vi "Command Engine.vi"(8 "error in (no error)":errorcluster, 10 "Parameters":T1 {"Compiled"."External Channels"."Channels" format="%.0x"; "Compiled"."External Channels"."Triggers" format="%.0x"}, 11 "Global Variables":T12) -> (0 "error out":errorcluster)   [LabVIEW 2015, in "Instrument Addon Engine.lvlib"]
uses:
  Instrument Addon Engine.lvlib
  Types/Engine State Variables.ctl
  <vilib>/NI/NIVS Inline Async API/_VS Inline Async API/Process/Process.lvclass
  <vilib>/NI/NIVS Addon Network Comm/Engine/VeriStand Comm.lvclass
  <vilib>/NI/NIVS Inline Async API/_Data Access Engine/Data Access Engine/Types/Write.DVR.ctl
  <vilib>/NI/NIVS Inline Async API/_Data Access Engine/Access Type Classes/Write/Write.lvclass
  <vilib>/NI/NIVS Inline Async API/_Data Access Engine/Data Access Engine/Types/Read.DVR.ctl
  <vilib>/NI/NIVS Inline Async API/_Data Access Engine/Access Type Classes/Read/Read.lvclass
  <vilib>/NI/NIVS Inline Async API/_Data Access Engine/Data Access Engine/Types/ReadWrite.DVR.ctl
  <vilib>/NI/NIVS Inline Async API/_Data Access Engine/Access Type Classes/ReadWrite/ReadWrite.lvclass
  Types/Commands RT Configuration Cluster.ctl
  Protocols.lvlibp/Protocol Parent/Protocol Parent.lvclass
  Shared/Types/Compiled Settings.ctl
  Shared/Types/Command Parameters.ctl
  Shared/Types/Linked Channel Cluster.ctl
  Shared/Types/Response RT Configuration Cluster.ctl
  Shared/Types/Response Parameters.ctl
  Shared/Types/Response Wait Type.ctl
  Shared/Types/Message Parameters.ctl
  Shared/Types/Message Generation Type.ctl
  Shared/Types/External Trigger Refs.ctl
  <vilib>/NI Veristand/Custom Device API/Data Reference.ctl
  Protections.lvlibp/Parent Protection/Protection.lvclass
  <vilib>/NI/NIVS Inline Async API/_Data Access Engine/Access Type Classes/ReadWrite/ReadWrite.lvclass/ReadWrite.ctl
  <vilib>/NI/NIVS Inline Async API/_Data Access Engine/Access Type Classes/Read/Read.lvclass/Read.ctl
  <vilib>/NI/NIVS Inline Async API/_Data Access Engine/Access Type Classes/Write/Write.lvclass/Write.ctl
  <vilib>/NI/NIVS Inline Async API/_VS Inline Async API/Process/Process.lvclass/Process.ctl
  Determine Trigger.vi
  <vilib>/NI/NIVS Inline Async API/_Data Access Engine/Data Access Engine/Methods/Data.Processes.Execute.vi
  <vilib>/NI/NIVS Inline Async API/_Data Access Engine/Data Access Engine/Methods/ReadWrite.Data.Read.vi
  <vilib>/NI/NIVS Inline Async API/_Data Access Engine/Data Access Engine/Methods/Read.Data.vi
  Format Instrument String Command.vi
  <vilib>/NI/NIVS Inline Async API/_Data Access Engine/Data Access Engine/Methods/Write.Data.vi
  <vilib>/NI/NIVS Inline Async API/_Data Access Engine/Data Access Engine/Methods/ReadWrite.Data.Reset.vi
  <vilib>/NI/NIVS Inline Async API/_VS Inline Async API/Error Handling Process/SubVIs/Error.ConvertArray.vi
  <vilib>/NI/NIVS Inline Async API/_Data Access Engine/Access Type Classes/ReadWrite/ReadWrite.ProcessData.Read.vi
  <vilib>/NI/NIVS Inline Async API/_Data Access Engine/Access Type Classes/Read/Read.ProcessData.vi
  Format Numeric to String.vi
  <vilib>/NI/NIVS Inline Async API/_Data Access Engine/Access Type Classes/Write/Write.ProcessData.vi
  <vilib>/NI/NIVS Inline Async API/_Data Access Engine/Access Type Classes/ReadWrite/ReadWrite.ProcessData.Reset.vi
  Get Wait Value from Channel.vi
  Send Instrument String Command.vi
  Wait on Instrument String Response.vi
  Format Instrument String Response.vi
  <vilib>/NI/AMC/AMC.lvlib
  Shared/Instrument Addon Shared.lvlib
  <vilib>/NI VeriStand/Custom Device API/Custom Device API.lvlib
  <vilib>/NI/NIVS Inline Async API/_Data Access Engine/Data Access Engine/Data Access Engine.lvclass
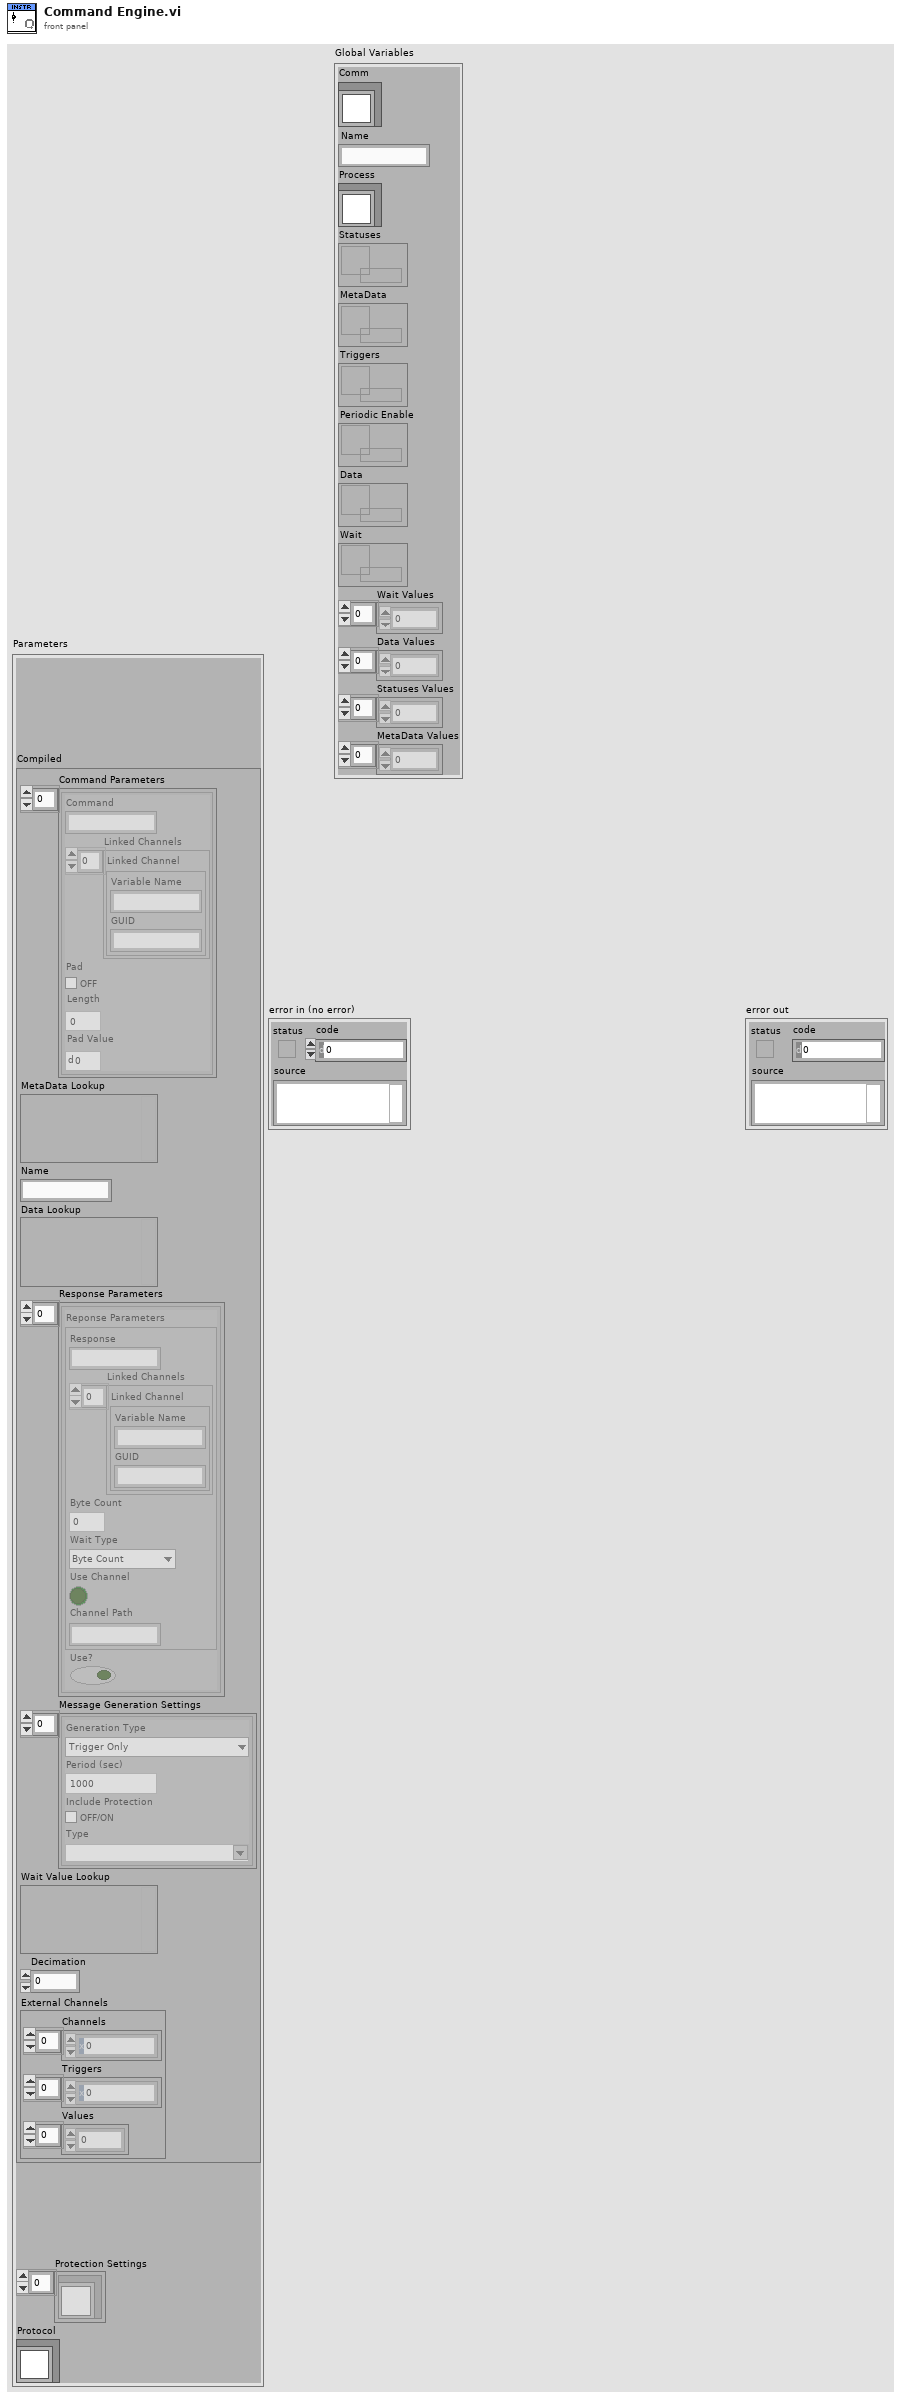
[diagram p1: front panel]
types:
  T1 = typedef "Instrument Addon Engine.lvlib/Commands RT Configuration Cluster.ctl" = cluster{"Compiled":T2, "Protection Settings":refnum<class "Protection.lvclass">[], "Protocol":refnum<class "Protocol Parent.lvclass">}
  T2 = typedef "Instrument Addon Shared.lvlib/Compiled Settings.ctl" = cluster{"Command Parameters":T3[], "MetaData Lookup":variant, "Name":string, "Data Lookup":variant, "Response Parameters":T5[], "Message Generation Settings":T8[], "Wait Value Lookup":variant, "Decimation":u32, "External Channels":T10}
  T3 = typedef "Instrument Addon Shared.lvlib/Command Parameters.ctl" = cluster{"Command":string, "Linked Channels":T4[], "Pad":bool, "Length":u32, "Pad Value":u8}
  T4 = typedef "Instrument Addon Shared.lvlib/Linked Channel Cluster.ctl" = cluster{"Variable Name":string, "GUID":string}
  T5 = typedef "Instrument Addon Shared.lvlib/Response RT Configuration Cluster.ctl" = cluster{"Reponse Parameters":T6, "Use?":bool}
  T6 = typedef "Instrument Addon Shared.lvlib/Response Parameters.ctl" = cluster{"Response":string, "Linked Channels":T4[], "Type Value":dbl, "Wait Type":T7, "Use Channel":bool, "Channel Path":string}
  T7 = typedef "Instrument Addon Shared.lvlib/Response Wait Type.ctl" = enum16{"Byte Count", "Wait sec"}
  T8 = typedef "Instrument Addon Shared.lvlib/Message Parameters.ctl" = cluster{"Generation Type":T9, "Period":dbl, "Include Protection":bool, "Type":string}
  T9 = typedef "Instrument Addon Shared.lvlib/Message Generation Type.ctl" = enum16{"Trigger Only", "Periodic & Trigger"}
  T10 = typedef "Instrument Addon Shared.lvlib/External Trigger Refs.ctl" = cluster{"Channels":T11[], "Triggers":T11[], "Values":dbl[]}
  T11 = typedef "Custom Device API.lvlib/Data Reference.ctl" = i32
  T12 = typedef "Instrument Addon Engine.lvlib/Engine State Variables.ctl" = cluster{"Comm":refnum<class "VeriStand Comm.lvclass">, "Name":string, "Process":refnum<class "Process.lvclass">, "Statuses":T13, "MetaData":T14, "Triggers":T15, "Periodic Enable":T14, "Data":T13, "Wait":T14, "Wait Values":dbl[], "Data Values":dbl[], "Statuses Values":dbl[], "MetaData Values":dbl[]}
  T13 = typedef "Data Access Engine.lvlib/Data Access Engine.lvclass/Write.DVR.ctl" = refnum<data-value>
  T14 = typedef "Data Access Engine.lvlib/Data Access Engine.lvclass/Read.DVR.ctl" = refnum<data-value>
  T15 = typedef "Data Access Engine.lvlib/Data Access Engine.lvclass/ReadWrite.DVR.ctl" = refnum<data-value>
  T16 = typedef "Instrument Addon Engine.lvlib/command engine global variables.ctl" = cluster{"Time":u32[], "Triggers":bool[], "Rsp Queue":T17, "# of Messages":i32, "Rsp Attributes":T18}
  T17 = typedef "AMC.lvlib/Message Queue.ctl" = refnum<queue>
  T18 = typedef "Tools_KeyedArray.lvlib/KeyedArray.ctl" = cluster{"keys":string[], "values":string[]}
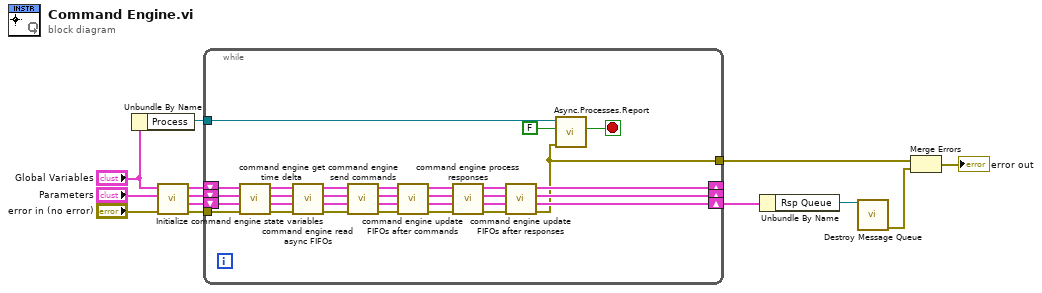
[diagram p0: block diagram]
diagram:
  n1 = Unbundle By Name("Global Variables") -> ("Process"=w13:refnum<class "Process.lvclass">)
  n2 = call "Initialize command engine state variables.vi"("error in (no error)"="error in (no error)", "Parameters"="Parameters", "Global Variables"="Global Variables") -> ("error out"=w10:errorcluster, "State Variables out"=w6:T16, "Parameters out"=w7:T1, "Global Variables out"=w8:T12)  [unwired: 5 in]
  n3 = while {
    tunnel: w10 -> [w41]
    tunnel: [w14] -> w3
    tunnel: w13 -> [w42]
    shift-right: [w23] -> _
    shift-left: w8 -> [w18]
    shift-right: [w22] -> _
    shift-left: w7 -> [w19]
    shift-right: [w21] -> w5
    shift-left: w6 -> [w20]
    stop <- w44 stop-if-true
    n4 = call "command engine get time delta.vi"("error in (no error)"=w41, "State Variables in"=w20, "Parameters"=w19, "Global Variables"=w18) -> ("error out"=w40:errorcluster, "State Variables out"=w16:T16, "Parameters out"=w17:T1, "Global Variables out"=w15:T12)  [unwired: 4 in]
    n5 = call "command engine read async FIFOs.vi"("error in (no error)"=w40, "State Variables"=w16, "Parameters"=w17, "Global Variables"=w15) -> ("error out"=w36:errorcluster, "State Variables out"=w38:T16, "Parameters out"=w37:T1, "Global Variables out"=w39:T12)  [unwired: 4 in]
    n6 = call "command engine send commands.vi"("error in (no error)"=w36, "State Variables"=w38, "Parameters"=w37, "Global Variables"=w39) -> ("error out"=w33:errorcluster, "State Variables out"=w34:T16, "Parameters out"=w35:T1, "Global Variables out"=w32:T12)  [unwired: 4 in]
    n7 = call "command engine update FIFOs after commands.vi"("error out"=w33, "State Variables in"=w34, "Parameters in"=w35, "Global Variables"=w32) -> ("error out"=w31:errorcluster, "State Variables out"=w30:T16, "Parameters out"=w29:T1, "Global Variables out"=w28:T12)  [unwired: 4 in]
    n8 = call "command engine process responses.vi"("error out"=w31, "State Variables"=w30, "Parameters"=w29, "Global Variables"=w28) -> ("error out"=w24:errorcluster, "State Variables out"=w25:T16, "Parameters out"=w27:T1, "Global Variables out"=w26:T12)  [unwired: 4 in]
    n9 = call "command engine update FIFOs after responses.vi"("error out"=w24, "State Variables in"=w25, "Parameters in"=w27, "Global Variables in"=w26) -> ("error out"=w14:errorcluster, "State Variables out"=w21:T16, "Parameters out"=w22:T1, "Global Variables out"=w23:T12)  [unwired: 4 in]
    n10 = call <vilib>:"Async.Processes.Report.vi"("Error"=w14, "Stop Async on Error?"=FALSE ("Stop on Error?"), "Process in"=w42) -> ("Stop"=w44:bool)  [unwired: 7 in, 1 out]
  }
  n11 = Unbundle By Name(w5) -> ("Rsp Queue"=w4:T17)
  n12 = call <vilib>:"Destroy Message Queue.vi"("message queue in"=w4) -> ("error out"=w2:errorcluster)  [unwired: 12 in, 2 out]
  n13 = Merge Errors(w3, w2) -> (→"error out":errorcluster)
